vi "NIconVert.vi"(0 "InstrumentID":refnum<k15>, 2 "V scale":T1 {"Coupling" items=["DC 1 MOhm", "AC 1 MOhm", "DC 50 Ohm", "AC 50 OHM"]; "Offset" format="%.2f"}, 3 "error in":errorcluster, 4 "Channel (0)":i32) -> (5 "Status":refnum<k15>, 7 "error out":errorcluster)   [LabVIEW 2022 SP3]
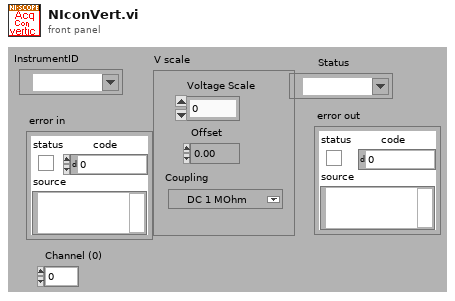
[diagram p1: front panel]
types:
  T1 = cluster{"Voltage Scale":dbl, "Offset":dbl, "Coupling":u16}
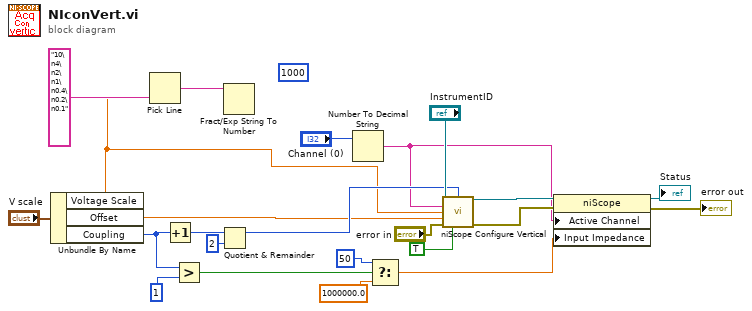
[diagram p0: block diagram]
diagram:
  (unwired) 1000
  n1 = Unbundle By Name("V scale") -> ("Voltage Scale"=w1:dbl, "Offset"=w4:dbl, "Coupling"=w8:u16)
  n2 = Pick Line(multi-line string="10\n4\n2\n1\n0.4\n0.2\n0.1", line index=w1) -> (output string=w21:string)  [unwired: 1 out]
  n3 = Increment(x=w8) -> (x+1=w13:u16)
  n4 = Greater?(x=w8, y=1) -> (0:w6:bool)
  n5 = Quotient & Remainder(x=w13, y=2) -> (x-y*floor(x/y)=w12:i32)  [unwired: 1 out]
  n6 = Fract/Exp String To Number(string=w21) -> ()  [unwired: 5 out]
  n7 = Number To Decimal String(number="Channel (0)") -> (decimal integer string=w2:string)  [unwired: 1 out]
  n8 = Select(t=50, s=w6, f=1000000.0) -> (s? t:f=w3:dbl)
  n9 = call <instrlib>:"niScope Configure Vertical.vi"("instrument handle"="InstrumentID", "vertical coupling"=w12, "channels"=w2, "vertical range"=w1, "vertical offset"=w4, "error in"="error in", "channel enabled"=TRUE) -> ("instrument handle out"=w18:refnum<k15>, "error out"=w17:errorcluster)  [unwired: 1 in, 6 out]
  n10 = property class="niScope"(reference=w18, error in=w17, "Active Channel"=w2, "Input Impedance"=w3) -> (reference out=→"Status":refnum<k15>, error out=→"error out":errorcluster)
